vi "myRIO_BRig_Host_plotCalc_minTrial.vi"(10 "input_maxTrialsDisplayed":i32, 11 "input_countTrial":i32) -> (3 "output_minTrial":i32)   [LabVIEW 2014]
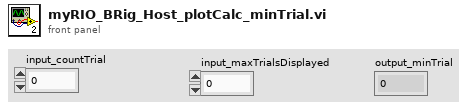
[diagram p1: front panel]
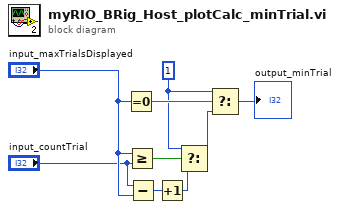
[diagram p0: block diagram]
diagram:
  w5 = 1 ("t")
  n1 = Equal To 0?(x="input_maxTrialsDisplayed") -> (x = 0?=w9:bool)
  n2 = Greater Or Equal?(x="input_maxTrialsDisplayed", y="input_countTrial") -> (x >= y?=w6:bool)
  n3 = Subtract(x="input_countTrial", y="input_maxTrialsDisplayed") -> (x-y=w2:i32)
  n4 = Increment(x=w2) -> (x+1=w1:i32)
  n5 = Select(t=w5, s=w6, f=w1) -> (s? t:f=w4:i32)
  n6 = Select(t=w5, s=w9, f=w4) -> (s? t:f=→"output_minTrial":i32)
